vi "Read Current Position.vi"(8 "error in (no error)":errorcluster, 11 "XY Stage Controller in":refnum<class "XY Stage Controller.lvclass">) -> (0 "error out":errorcluster, 1 "Y Position":dbl, 2 "X Position":dbl, 3 "XY Stage Controller out":refnum<class "XY Stage Controller.lvclass">)   [LabVIEW 2022 SP3, in "XY Stage Controller.lvclass"]
uses:
  XY Stage Controller.lvclass
  XY Stage Controller.lvclass/XY Stage Controller.ctl
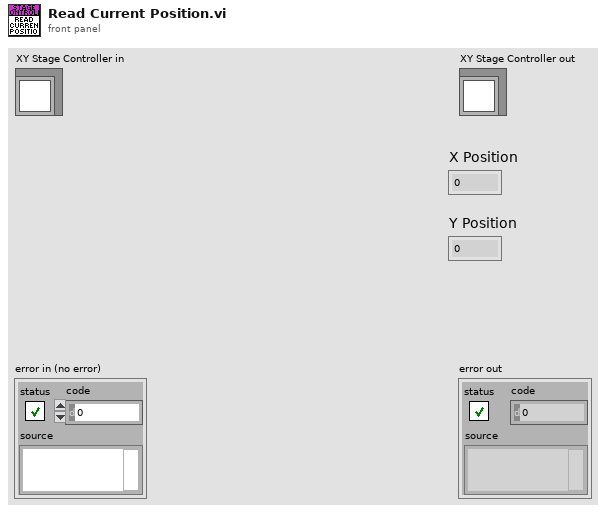
[diagram p1: front panel]
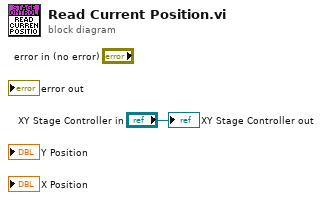
[diagram p0: block diagram]
diagram:
  "XY Stage Controller out" <- "XY Stage Controller in"
